vi "UMLEditor ScriptRemoveMethodsValidator.vi"(0 "RefnumIn":T1, 5 "error in (no error)":errorcluster, 6 "ClassSection":string="ClassFolder") -> (14 "RefnumOut":T1, 19 "error out":errorcluster)   [LabVIEW 2016]
uses:
  <vilib>/Utility/config.llb/Config Data RefNum.ctl
  <vilib>/Utility/config.llb/Read Key (String).vi
  <vilib>/Utility/config.llb/Write Key (String).vi
  <vilib>/Utility/config.llb/NI_LVConfig.lvlib
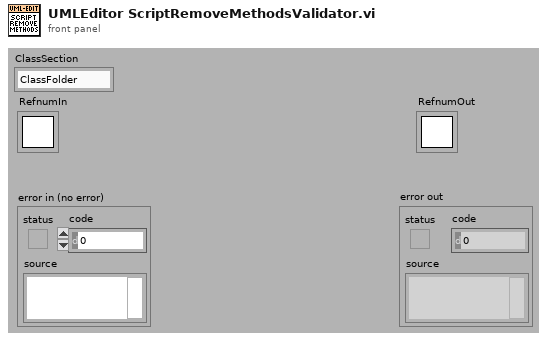
[diagram p1: front panel]
types:
  T1 = typedef "NI_LVConfig.lvlib/Config Data RefNum.ctl" = refnum<k1>
  T2 = cluster{"RemovedMethods":i32[], "size":i32, "Methods":i32[]}
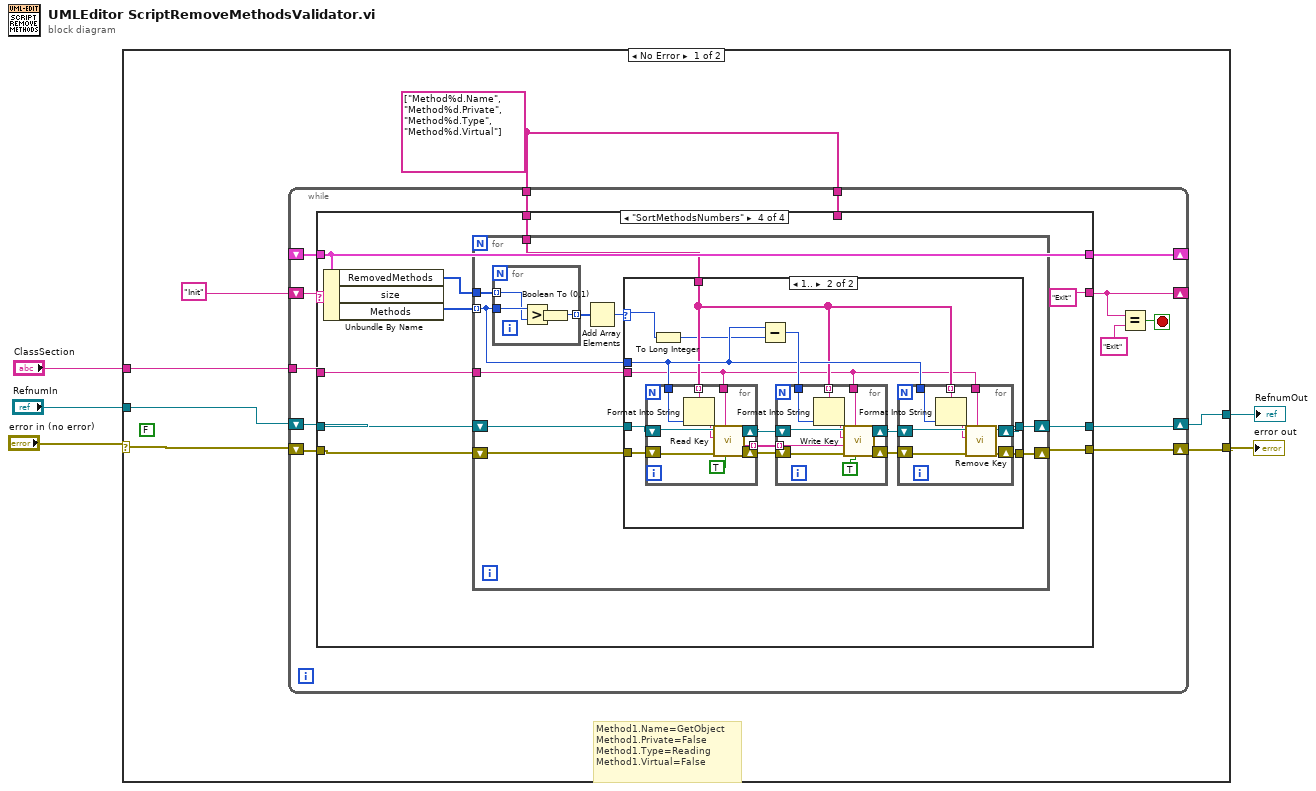
[diagram p0: block diagram]
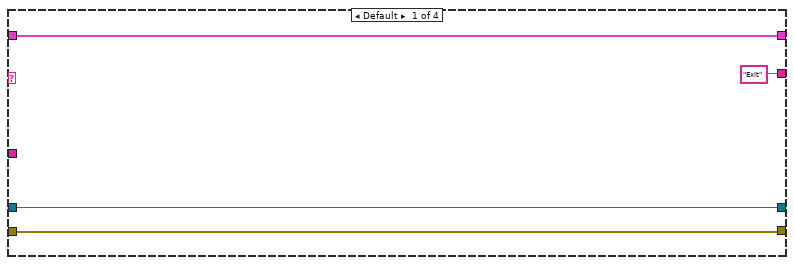
[diagram p2: hidden frame]
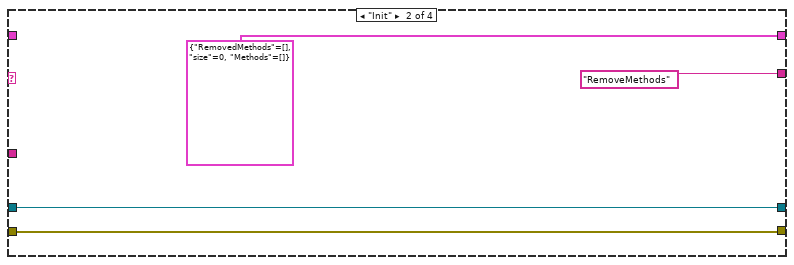
[diagram p3: hidden frame]
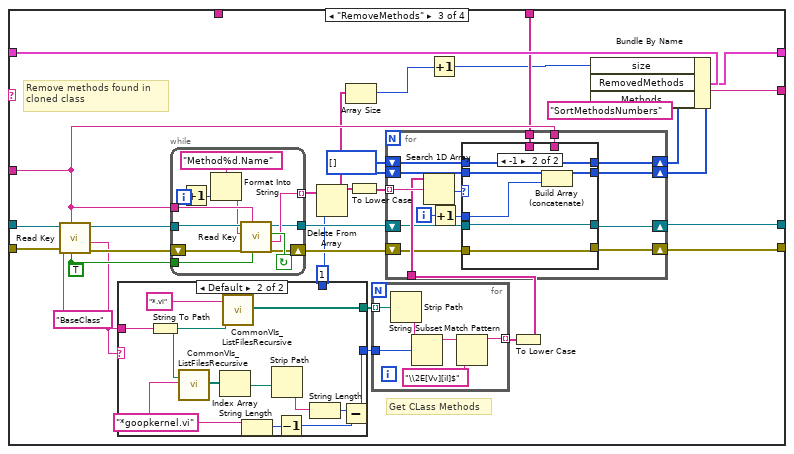
[diagram p4: hidden frame]
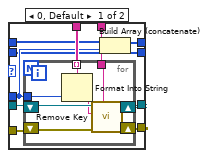
[diagram p6: hidden frame]
diagram:
  n1 = case shown="No Error" "error in (no error)" {
    selector: "error in (no error)" -> [w11 w203]
    tunnel: [w9 w203] -> w4
    tunnel: "RefnumIn" -> [w12 w202]
    tunnel: "ClassSection" -> [w10 _]
    tunnel: [w6 w202] -> w1
    frame No Error {
      w7 = string[] ["Method%d.Name", "Method%d.Private", "Method%d.Type", "Method%d.Virtual"]
      (unwired) FALSE ("create file if necessary? (T)")
      # "Method1.Name=GetObject\nMethod1.Private=False\nMethod1.Type=Reading\nMethod1.Virtual=False"
      n2 = while {
        shift-right: [w25] -> w9
        shift-left: w11 -> [w22]
        shift-right: [w24] -> w6
        shift-left: w12 -> [w23]
        tunnel: w10 -> [w21]
        shift-right: [w15] -> _
        shift-left: "Init" -> [w20]
        shift-right: [w18] -> _
        shift-left: _ -> [w19]
        tunnel: w7 -> [w17]
        tunnel: w7 -> [w16]
        stop <- w13 stop-if-true
        n3 = case shown="\"SortMethodsNumbers\"" w20 {
          tunnel: w23 -> [w29 w31 w62 w138]
          tunnel: w22 -> [w28 w30 w61 w137]
          tunnel: w21 -> [_ _ w53 w141]
          tunnel: [w29 w31 w47 w135] -> w24
          tunnel: [w28 w30 w48 w136] -> w25
          tunnel: ["Exit" ("FileSearchPattern") "RemoveMethods" "SortMethodsNumbers" ("FileSearchPattern") "Exit" ("FileSearchPattern")] -> w15
          tunnel: w19 -> [w26 _ w45 w133]
          tunnel: [w26 T2 {"RemovedMethods"=[], "size"=0, "Methods"=[]} w44 w133] -> w18
          tunnel: w17 -> [_ _ w42 _]
          tunnel: w16 -> [_ _ _ w142]
          frame Default {
          }
          frame "Init" {
          }
          frame "RemoveMethods" {
            w36 = i32[] []
            w55 = TRUE ("read raw string? (F)")
            # "Get CLass Methods"
            # "Remove methods found in\ncloned class"
            n4 = call-poly <vilib>:"Read Key.vi"("read raw string? (F)"=w55, "section"=w53, "error in (no error)"=w61, "key"="BaseClass", "refnum"=w62) -> ("error out"=w57:errorcluster, "value"=w34:string, "refnum out"=w56:T1)  [unwired: 1 in, 3 out]
            n5 = case shown="Default" w34 {
              tunnel: w34 -> [_ w75]
              tunnel: [_ w67] -> w59
              tunnel: [_ w66] -> w58
              tunnel: [_ 1 ("length")] -> w40
              frame "" {
              }
              frame Default {
                w69 = "*goopkernel.vi" ("FileSearchPattern")
                n6 = String To Path(string=w75) -> (path=w73:path)
                n7 = call <resource>:"CommonVIs_ListFilesRecursive.vi"("directory path"=w73, "FileSearchPattern"=w69) -> ("Files"=w72:path[])  [unwired: 4 in, 13 out]
                n8 = Index Array(array=w72) -> (element=w65:path)  [unwired: 1 in]
                n9 = call <resource>:"CommonVIs_ListFilesRecursive.vi"("directory path"=w73, "FileSearchPattern"="*.vi") -> ("Files"=w67:path[])  [unwired: 4 in, 13 out]
                n10 = String Length(string=w69) -> (length=w70:i32)
                n11 = Strip Path(path=w65) -> (name=w64:string)  [unwired: 1 out]
                n12 = Decrement(x=w70) -> (x-1=w68:i32)
                n13 = String Length(string=w64) -> (length=w71:i32)
                n14 = Subtract(x=w71, y=w68) -> (x-y=w66:i32)
              }
            }
            n15 = while {
              shift-right: [w116] -> w49
              shift-left: w57 -> [w126]
              tunnel: w56 -> [w125]
              tunnel: w53 -> [w124]
              tunnel: w55 -> [w119]
              tunnel: [w117] -> w41 mode=indexing
              tunnel: [w115] -> w50
              i -> [w122]
              stop <- w118 continue-if-true
              n16 = Increment(x=w122) -> (x+1=w121:i32)
              n17 = Format Into String(format string="Method%d.Name", w121) -> (resulting string=w120:string)  [unwired: 2 in, 1 out]
              n18 = call-poly <vilib>:"Read Key.vi"("read raw string? (F)"=w119, "section"=w124, "error in (no error)"=w126, "key"=w120, "refnum"=w125) -> ("error out"=w116:errorcluster, "value"=w117:string, "found?"=w118:bool, "refnum out"=w115:T1)  [unwired: 1 in, 2 out]
            }
            n19 = Delete From Array(array=w41, length=w40) -> (array with subset deleted=w39:string[])  [unwired: 1 in, 1 out]
            n20 = Array Size(array=w39) -> (size(s)=w38:i32)
            n21 = To Lower Case(string=w39) -> (all lower case string=w52:string[])
            n22 = for {
              tunnel: w59 -> [w132] mode=indexing
              tunnel: w58 -> [w130]
              tunnel: [w127] -> w54 mode=indexing
              n23 = Strip Path(path=w132) -> (name=w131:string)  [unwired: 1 out]
              n24 = String Subset(string=w131, offset (0)=w130) -> (substring=w129:string)  [unwired: 1 out]
              n25 = Match Pattern(string=w129, regular expression="\\2E[Vv][iI]$") -> (before substring=w127:string)  [unwired: 4 out]
            }
            n26 = Increment(x=w38) -> (x+1=w37:i32)
            n27 = To Lower Case(string=w54) -> (all lower case string=w51:string[])
            n28 = for {
              tunnel: w53 -> [w90]
              tunnel: w42 -> [w89]
              tunnel: w52 -> [w88] mode=indexing
              tunnel: w51 -> [w87]
              shift-right: [w82] -> w48
              shift-left: w49 -> [w85]
              shift-right: [w83] -> w47
              shift-left: w50 -> [w84]
              shift-right: [w81] -> w43
              shift-left: w36 -> [w80]
              shift-right: [w76] -> w35
              shift-left: w36 -> [w77]
              i -> [w79]
              n29 = Search 1D Array(1D array=w87, element=w88) -> (index of element=w86:i32)  [unwired: 1 out]
              n30 = Increment(x=w79) -> (x+1=w78:i32)
              n31 = case shown="-1" w86 {
                tunnel: w90 -> [w100 _]
                tunnel: w89 -> [w99 _]
                tunnel: [w98 w114] -> w83
                tunnel: [w97 w113] -> w82
                tunnel: w85 -> [w96 w113]
                tunnel: w84 -> [w95 w114]
                tunnel: w78 -> [w92 w109]
                tunnel: [w94 w112] -> w81
                tunnel: w80 -> [w93 w112]
                tunnel: w77 -> [w91 w111]
                tunnel: [w91 w110] -> w76
                frame 0, Default {
                  n32 = for {
                    shift-right: [w103] -> w98
                    shift-left: w95 -> [w108]
                    shift-right: [w104] -> w97
                    shift-left: w96 -> [w107]
                    tunnel: w100 -> [w106]
                    tunnel: w99 -> [w105] mode=indexing
                    tunnel: w92 -> [w101]
                    n33 = Format Into String(format string=w105, w101) -> (resulting string=w102:string)  [unwired: 2 in, 1 out]
                    n34 = call <vilib>:"Remove Key.vi"("section"=w106, "error in (no error)"=w107, "key"=w102, "refnum"=w108) -> ("error out"=w104:errorcluster, "refnum out"=w103:T1)  [unwired: 6 out]
                  }
                  n35 = Build Array (concatenate)(w93, w92) -> (w94:i32[])
                }
                frame -1 {
                  n36 = Build Array (concatenate)(w111, w109) -> (w110:i32[])
                }
              }
            }
            n37 = Bundle By Name(cluster=w45, "size"=w37, "RemovedMethods"=w43, "Methods"=w35) -> (w44:T2)
          }
          frame "SortMethodsNumbers" {
            n38 = Unbundle By Name(w133) -> ("RemovedMethods"=w139:i32[], "Methods"=w140:i32[])  [unwired: 1 out]
            n39 = for {
              tunnel: w142 -> [w152]
              tunnel: w141 -> [w151]
              tunnel: w140 -> [w148] mode=indexing
              tunnel: w139 -> [w150]
              shift-right: [w144] -> w136
              shift-left: w137 -> [w145]
              shift-right: [w143] -> w135
              shift-left: w138 -> [w146]
              n40 = for {
                tunnel: w148 -> [w201]
                tunnel: w150 -> [w200] mode=indexing
                tunnel: [w198] -> w149 mode=indexing
                n41 = Greater?(x=w201, y=w200) -> (0:w199:bool)
                n42 = Boolean To (0,1)(Boolean=w199) -> (0, 1=w198:i16)
              }
              n43 = Add Array Elements(numeric array=w149) -> (sum=w147:i16)
              n44 = case shown="1.." w147 {
                selector: w147 -> [_ w166]
                tunnel: w145 -> [w153 w169]
                tunnel: w146 -> [w154 w168]
                tunnel: w152 -> [_ w160]
                tunnel: w151 -> [_ w159]
                tunnel: w148 -> [_ w161]
                tunnel: [w153 w158] -> w144
                tunnel: [w154 w157] -> w143
                frame 0, Default {
                }
                frame 1.. {
                  n45 = for {
                    shift-right: [w192] -> w156
                    shift-left: w168 -> [w197]
                    shift-right: [w193] -> w167
                    shift-left: w169 -> [w196]
                    tunnel: w159 -> [w195]
                    tunnel: w160 -> [w194] mode=indexing
                    tunnel: w161 -> [w188]
                    tunnel: [w189] -> w162 mode=indexing
                    n46 = Format Into String(format string=w194, w188) -> (resulting string=w191:string)  [unwired: 2 in, 1 out]
                    n47 = call-poly <vilib>:"Read Key.vi"("read raw string? (F)"=TRUE, "section"=w195, "error in (no error)"=w196, "key"=w191, "refnum"=w197) -> ("error out"=w193:errorcluster, "value"=w189:string, "refnum out"=w192:T1)  [unwired: 1 in, 3 out]
                  }
                  n48 = To Long Integer(number=w166) -> (32bit integer=w155:i32)
                  n49 = Subtract(x=w161, y=w155) -> (x-y=w165:i32)
                  n50 = for {
                    shift-right: [w182] -> w164
                    shift-left: w156 -> [w187]
                    shift-right: [w183] -> w163
                    shift-left: w167 -> [w186]
                    tunnel: w159 -> [w185]
                    tunnel: w160 -> [w184] mode=indexing
                    tunnel: w165 -> [w178]
                    tunnel: w162 -> [w179] mode=indexing
                    n51 = Format Into String(format string=w184, w178) -> (resulting string=w181:string)  [unwired: 2 in, 1 out]
                    n52 = call-poly <vilib>:"Write Key.vi"("write raw string? (F)"=TRUE ("read raw string? (F)"), "section"=w185, "error in (no error)"=w186, "value"=w179, "key"=w181, "refnum"=w187) -> ("error out"=w183:errorcluster, "refnum out"=w182:T1)  [unwired: 4 out]
                  }
                  n53 = for {
                    shift-right: [w172] -> w157
                    shift-left: w164 -> [w177]
                    shift-right: [w173] -> w158
                    shift-left: w163 -> [w176]
                    tunnel: w159 -> [w175]
                    tunnel: w160 -> [w174] mode=indexing
                    tunnel: w161 -> [w170]
                    n54 = Format Into String(format string=w174, w170) -> (resulting string=w171:string)  [unwired: 2 in, 1 out]
                    n55 = call <vilib>:"Remove Key.vi"("section"=w175, "error in (no error)"=w176, "key"=w171, "refnum"=w177) -> ("error out"=w173:errorcluster, "refnum out"=w172:T1)  [unwired: 1 in, 5 out]
                  }
                }
              }
            }
          }
        }
        n56 = Equal?(x=w15, y="Exit" ("FileSearchPattern")) -> (x = y?=w13:bool)
      }
    }
    frame Error {
    }
  }
  "error out" <- w4
  "RefnumOut" <- w1
